vi "Teleop.vi"(10 "Match Info":T1={"Autonomous Elapsed Seconds"=0.0, "TeleOp Elapsed Seconds"=0.0, "Disabled Elapsed Seconds"=0.0, "Visited Autonomous"=FALSE, "Visited TeleOp"=FALSE, "Visited Disabled"=FALSE, "Autonomous Settings"={"Autonomous Style"=enum."Independent", "VI Refnum"=refnum}}, 11 "Call Context":T2) -> ()   [LabVIEW 2012]
doc: "This VI is called for each TeleOp packet received from the DS where the robot is not disabled. It is often used to read from the joysticks and update I/O or to update setpoints for timed control loops. It should complete and return within 20 milliseconds or it may miss DS packets."
uses:
  <vilib>/Rock Robotics/WPI/DriverStation/WPI_DriverStationDerivedRobotMode.ctl
  <vilib>/Rock Robotics/WPI/DriverStation/WPI_DriverStationMatch Info.ctl
  Robot Global Data.vi
  <vilib>/Rock Robotics/WPI/Joystick/WPI_JoystickGetSetRefNum.vi
  <vilib>/Rock Robotics/WPI/RobotDrive/WPI_RobotDriveGetSetRefNum.vi
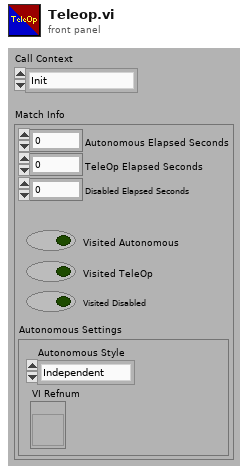
[diagram p1: front panel]
types:
  T1 = typedef "WPI_DriverStationMatch Info.ctl" = cluster{"Autonomous Elapsed Seconds":dbl, "TeleOp Elapsed Seconds":dbl, "Disabled Elapsed Seconds":dbl, "Visited Autonomous":bool, "Visited TeleOp":bool, "Visited Disabled":bool, "Autonomous Settings":cluster{"Autonomous Style":enum16{"Iterative", "Independent"}, "VI Refnum":refnum<vi>}}
  T2 = typedef "WPI_DriverStationDerivedRobotMode.ctl" = enum16{"Init", "Execute", "Stop"}
  T3 = typedef "WPI_DigitalInputDevRef.ctl" = cluster{"DevStatus":errorcluster, "DIO Channel":T4, "Digital Module":T5}
  T4 = typedef "FPGA_DIOChannel.ctl" = enum8{"DIO 1", "DIO 2", "DIO 3", "DIO 4", "DIO 5", "DIO 6", "DIO 7", "DIO 8", "DIO 9", "DIO 10", "DIO 11", "DIO 12", "DIO 13", "DIO 14", "Invalid"}
  T5 = typedef "FPGA_TypedefDigitalModule.ctl" = enum16{"Digital Module 1", "Digital Module 2"}
  T6 = cluster{"Prox1":bool, "Prox2":bool, "Prox3":bool, "Frisbee_Catch":bool, "Frisbee_Side_Check":bool, "Shooter_Ready":bool, "LeadScrewEnd":bool}
  T7 = typedef "WPI_JoystickDevRef.ctl" = cluster{"Device":T8}
  T8 = typedef "WPI_JoystickDeviceEnum.ctl" = enum16{"USB 1", "USB 2", "USB 3", "USB 4", "Kinect 1", "Kinect 2"}
  T9 = typedef "WPI_JoystickButtonState.ctl" = cluster{"Button 1":bool, "Button 2":bool, "Button 3":bool, "Button 4":bool, "Button 5":bool, "Button 6":bool, "Button 7":bool, "Button 8":bool, "Button 9":bool, "Button 10":bool, "Button 11":bool, "Button 12":bool}
  T10 = cluster{"axis 1 (x)":dbl, "axis 2 (y)":dbl, "axis 3 (throttle)":dbl, "axis 4":dbl, "axis 5":dbl, "axis 6":dbl}
  T11 = typedef "WPI_RobotDriveDevRef.ctl" = cluster{"DevStatus":errorcluster, "Motors[]":T12[], "Square Inputs":bool, "Max Output":dbl, "Isochronous":bool}
  T12 = typedef "WPI_MotorControlDeviceRef.ctl" = cluster{"DeviceStatus":errorcluster, "Type":enum16{"PWM", "CAN"}, "PWM":cluster{"Digital Module":T5, "PWM Channel":T13, "DeadBand":T14}, "CAN":cluster{"Device Number":u8, "Control Mode":T15, "Semaphore":T16, "Max Vout":dbl}, "Invert":bool, "TransformRef":T17, "InvTransformRef":T17}
  T13 = typedef "FPGA_DIOPWMChannel.ctl" = enum8{"PWM 1", "PWM 2", "PWM 3", "PWM 4", "PWM 5", "PWM 6", "PWM 7", "PWM 8", "PWM 9", "PWM 10", "Invalid"}
  T14 = typedef "WPI_PWMDeadband.ctl" = cluster{"Name":string, "maxPositivePwm":i32, "minPositivePwm":i32, "centerPwm":i32, "maxNegativePwm":i32, "minNegativePwm":i32, "angularRange":u16}
  T15 = typedef "WPI_CANJaguar_ControlMode.ctl" = enum8{"Percent VBus", "Current", "Speed", "Position", "Voltage"}
  T16 = typedef "Semaphore RefNum" = refnum<k1>
  T17 = typedef "WPI_PWMTransform_ConPane.ctl" = refnum<vi>
  T18 = cluster{"Shoot":bool, "Enable_Targeting":bool, "Shooter":dbl, "LeadScrew":dbl, "Feed":bool, "SuctionCup":bool, "SuctionRotate":bool, "SuctionExtend":bool, "Pickup":bool, "PizzaBottom":bool, "PizzaMid":bool, "Pizza_top":bool}
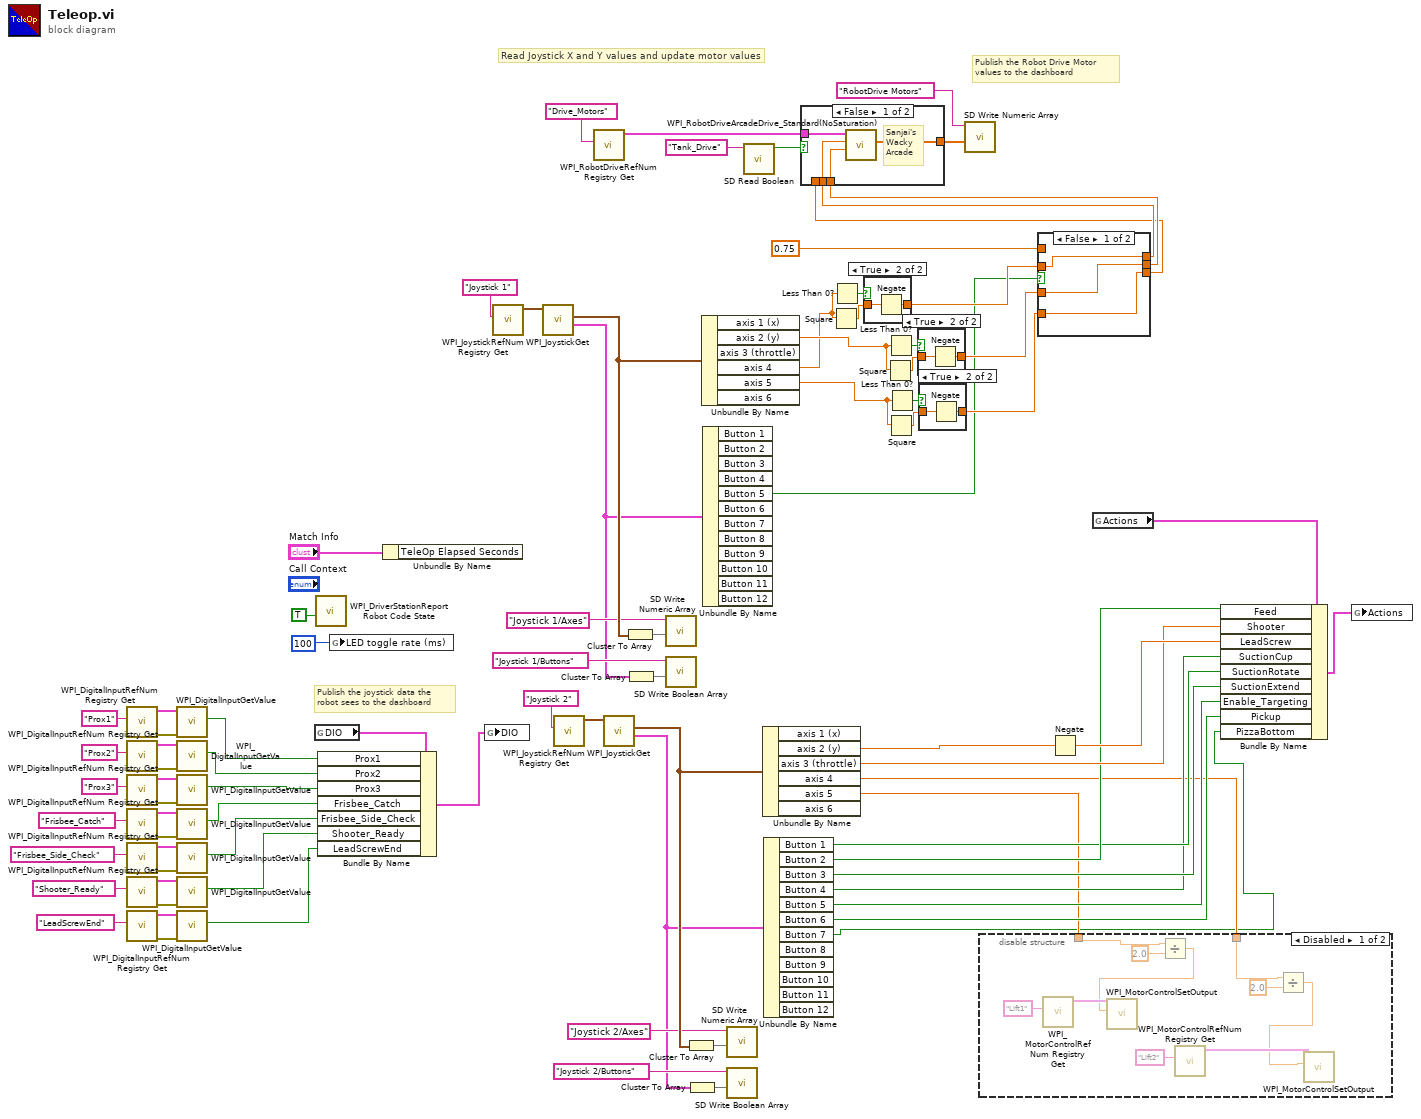
[diagram p0: block diagram]
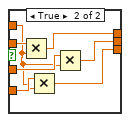
[diagram p3: hidden frame]
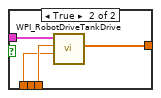
[diagram p7: hidden frame]
diagram:
  # "Publish the Robot Drive Motor\nvalues to the dashboard"
  # "Publish the joystick data the\nrobot sees to the dashboard"
  # "Read Joystick X and Y values and update motor values"
  n1 = call <vilib>:"WPI_DigitalInputRefNum Registry Get.vi"("refnum name"="Prox1") -> ("error out"=w61:errorcluster, "DigitalInputDevRef"=w60:T3)  [unwired: 9 in]
  n2 = call <vilib>:"WPI_DigitalInputRefNum Registry Get.vi"("refnum name"="Prox2") -> ("error out"=w52:errorcluster, "DigitalInputDevRef"=w53:T3)  [unwired: 9 in]
  n3 = call <vilib>:"WPI_DigitalInputRefNum Registry Get.vi"("refnum name"="Prox3") -> ("error out"=w51:errorcluster, "DigitalInputDevRef"=w54:T3)  [unwired: 9 in]
  n4 = call <vilib>:"WPI_DigitalInputRefNum Registry Get.vi"("refnum name"="Frisbee_Catch") -> ("error out"=w50:errorcluster, "DigitalInputDevRef"=w55:T3)  [unwired: 9 in]
  n5 = call <vilib>:"WPI_DigitalInputRefNum Registry Get.vi"("refnum name"="Frisbee_Side_Check") -> ("error out"=w57:errorcluster, "DigitalInputDevRef"=w56:T3)  [unwired: 9 in]
  n6 = call <vilib>:"WPI_DigitalInputRefNum Registry Get.vi"("refnum name"="Shooter_Ready") -> ("error out"=w59:errorcluster, "DigitalInputDevRef"=w58:T3)  [unwired: 9 in]
  n7 = call <vilib>:"WPI_DigitalInputRefNum Registry Get.vi"("refnum name"="LeadScrewEnd") -> ("error out"=w17:errorcluster, "DigitalInputDevRef"=w16:T3)  [unwired: 9 in]
  n8 = call <vilib>:"WPI_DigitalInputGetValue.vi"("error in (no error)"=w61, "DigitalInputDevRef"=w60) -> ("Value"=w44:bool)  [unwired: 7 in, 2 out]
  n9 = call <vilib>:"WPI_DigitalInputGetValue.vi"("error in (no error)"=w52, "DigitalInputDevRef"=w53) -> ("Value"=w49:bool)  [unwired: 7 in, 2 out]
  n10 = call <vilib>:"WPI_DigitalInputGetValue.vi"("error in (no error)"=w51, "DigitalInputDevRef"=w54) -> ("Value"=w48:bool)  [unwired: 7 in, 2 out]
  n11 = call <vilib>:"WPI_DigitalInputGetValue.vi"("error in (no error)"=w50, "DigitalInputDevRef"=w55) -> ("Value"=w47:bool)  [unwired: 7 in, 2 out]
  n12 = call <vilib>:"WPI_DigitalInputGetValue.vi"("error in (no error)"=w57, "DigitalInputDevRef"=w56) -> ("Value"=w46:bool)  [unwired: 7 in, 2 out]
  n13 = call <vilib>:"WPI_DigitalInputGetValue.vi"("error in (no error)"=w59, "DigitalInputDevRef"=w58) -> ("Value"=w45:bool)  [unwired: 7 in, 2 out]
  n14 = call <vilib>:"WPI_DigitalInputGetValue.vi"("error in (no error)"=w17, "DigitalInputDevRef"=w16) -> ("Value"=w14:bool)  [unwired: 7 in, 2 out]
  n15 = global read "Robot Global Data.vi" "DIO"() -> (w69:T6)
  n16 = call <vilib>:"WPI_DriverStationReport Robot Code State.vi"("TeleOp"=TRUE ("Autonomous")) -> ()  [unwired: 10 in, 1 out]
  n17 = Bundle By Name(cluster=w69, "Prox1"=w44, "Prox2"=w49, "Prox3"=w48, "Frisbee_Catch"=w47, "Frisbee_Side_Check"=w46, "Shooter_Ready"=w45, "LeadScrewEnd"=w14) -> (w68:T6)
  n18 = global write "Robot Global Data.vi" "LED toggle rate (ms)"(u32 100 ("LED ms toggle rate")) -> ()
  n19 = Unbundle By Name("Match Info") -> ()  [unwired: 1 out]
  n20 = global write "Robot Global Data.vi" "DIO"(w68) -> ()
  n21 = call <vilib>:"WPI_JoystickRefNum Registry Get.vi"("refnum name"="Joystick 1") -> ("JoystickDevRef"=w81:T7)  [unwired: 1 in, 9 out]
  n22 = call <vilib>:"WPI_JoystickGet.vi"("JoystickDevRef"=w81) -> ("Buttons"=w71:T9, "Axes"=w78:T10)  [unwired: 1 in, 4 out]
  n23 = call <vilib>:"WPI_JoystickRefNum Registry Get.vi"("refnum name"="Joystick 2") -> ("JoystickDevRef"=w34:T7)  [unwired: 1 in, 9 out]
  n24 = call <vilib>:"WPI_RobotDriveRefNum Registry Get.vi"("refnum name"="Drive_Motors") -> ("RobotDriveDevRef"=w83:T11)  [unwired: 1 in, 9 out]
  n25 = call <vilib>:"WPI_JoystickGet.vi"("JoystickDevRef"=w34) -> ("Buttons"=w28:T9, "Axes"=w31:T10)  [unwired: 1 in, 4 out]
  n26 = Cluster To Array(cluster=w78) -> (array=w77:dbl[])
  n27 = Cluster To Array(cluster=w71) -> (array=w80:bool[])
  n28 = call <vilib>:"SD Write Numeric Array.vi"("Numeric Array"=w77, "Name"="Joystick 1/Axes") -> ()  [unwired: 8 in, 2 out]
  n29 = call <vilib>:"SD Write Boolean Array.vi"("Boolean Array"=w80, "Name"="Joystick 1/Buttons") -> ()  [unwired: 8 in, 2 out]
  n30 = Cluster To Array(cluster=w31) -> (array=w30:dbl[])
  n31 = Cluster To Array(cluster=w28) -> (array=w33:bool[])
  n32 = Unbundle By Name(w78) -> ("axis 2 (y)"=w39:dbl, "axis 4"=w36:dbl, "axis 5"=w35:dbl)  [unwired: 3 out]
  n33 = Unbundle By Name(w71) -> ("Button 5"=w19:bool)  [unwired: 11 out]
  n34 = call <vilib>:"SD Write Numeric Array.vi"("Numeric Array"=w30, "Name"="Joystick 2/Axes") -> ()  [unwired: 8 in, 2 out]
  n35 = call <vilib>:"SD Write Boolean Array.vi"("Boolean Array"=w33, "Name"="Joystick 2/Buttons") -> ()  [unwired: 8 in, 2 out]
  n36 = call <vilib>:"SD Read Boolean.vi"("Name"="Tank_Drive") -> ("Boolean"=w73:bool)  [unwired: 8 in, 2 out]
  n37 = Unbundle By Name(w31) -> ("axis 2 (y)"=w15:dbl, "axis 3 (throttle)"=w10:dbl, "axis 4"=w3:dbl, "axis 5"=w2:dbl)  [unwired: 2 out]
  n38 = Unbundle By Name(w28) -> ("Button 1"=w7:bool, "Button 2"=w9:bool, "Button 3"=w8:bool, "Button 4"=w6:bool, "Button 5"=w5:bool, "Button 6"=w4:bool, "Button 7"=w1:bool)  [unwired: 5 out]
  n39 = Square(x=w36) -> (x^2=w43:dbl)
  n40 = Less Than 0?(x=w36) -> (x < 0?=w42:bool)
  n41 = case shown="True" w42 {
    tunnel: [w87 w88] -> w24
    tunnel: w43 -> [w87 w89]
    frame False {
    }
    frame True {
      n42 = Negate(x=w89) -> (-x=w88:dbl)
    }
  }
  n43 = Square(x=w39) -> (x^2=w41:dbl)
  n44 = Less Than 0?(x=w39) -> (x < 0?=w40:bool)
  n45 = Square(x=w35) -> (x^2=w38:dbl)
  n46 = Less Than 0?(x=w35) -> (x < 0?=w37:bool)
  n47 = case shown="True" w40 {
    tunnel: [w90 w91] -> w26
    tunnel: w41 -> [w90 w92]
    frame False {
    }
    frame True {
      n48 = Negate(x=w92) -> (-x=w91:dbl)
    }
  }
  n49 = case shown="True" w37 {
    tunnel: [w93 w94] -> w25
    tunnel: w38 -> [w93 w95]
    frame False {
    }
    frame True {
      n50 = Negate(x=w95) -> (-x=w94:dbl)
    }
  }
  n51 = disable-structure shown="Disabled" {
    disable-tunnel: w3 -> [w101 _]
    disable-tunnel: w2 -> [w97 _]
    frame Disabled {
      n52 = call <vilib>:"WPI_MotorControlRefNum Registry Get.vi"("refnum name"="Lift1") -> ("MotorControlDevRef"=w105:T12)  [unwired: 9 in, 1 out]
      n53 = Divide(x=w97, y=2.0) -> (x/y=w96:dbl)
      n54 = call <vilib>:"WPI_MotorControlSetOutput.vi"("Output"=w96, "MotorControlDevRef"=w105) -> ()  [unwired: 7 in, 3 out]
      n55 = call <vilib>:"WPI_MotorControlRefNum Registry Get.vi"("refnum name"="Lift2") -> ("MotorControlDevRef"=w103:T12)  [unwired: 9 in, 1 out]
      n56 = Divide(x=w101, y=2.0) -> (x/y=w99:dbl)
      n57 = call <vilib>:"WPI_MotorControlSetOutput.vi"("Output"=w99, "MotorControlDevRef"=w103) -> ()  [unwired: 7 in, 3 out]
    }
    frame Enabled {
    }
  }
  n58 = case shown="False" w19 {
    tunnel: w26 -> [w106 w115]
    tunnel: w25 -> [w107 w114]
    tunnel: w24 -> [w108 w113]
    tunnel: [w108 w110] -> w22
    tunnel: [w106 w112] -> w23
    tunnel: [w107 w111] -> w21
    tunnel: 0.75 -> [_ w109]
    frame False {
    }
    frame True {
      n59 = Multiply(x=w113, y=w109) -> (x*y=w110:dbl)
      n60 = Multiply(x=w114, y=w109) -> (x*y=w111:dbl)
      n61 = Multiply(x=w115, y=w109) -> (x*y=w112:dbl)
    }
  }
  n62 = case shown="False" w73 {
    tunnel: w83 -> [w119 w122]
    tunnel: [w118 w123] -> w74
    tunnel: w22 -> [w117 _]
    tunnel: w23 -> [w116 w121]
    tunnel: w21 -> [_ w120]
    frame False {
      # "Sanjai's\nWacky\nArcade"
      n63 = call <vilib>:"WPI_RobotDriveArcadeDrive_Standard(NoSaturation).vi"("Y axis value"=w116, "X axis value"=w117, "RobotDriveDevRef"=w119) -> ("Motor Values"=w118:dbl[])  [unwired: 1 in, 7 out]
    }
    frame True {
      n64 = call <vilib>:"WPI_RobotDriveTankDrive.vi"("Right axis value"=w120, "Left axis value"=w121, "RobotDriveDevRef"=w122) -> ("Motor Values"=w123:dbl[])  [unwired: 6 in, 2 out]
    }
  }
  n65 = call <vilib>:"SD Write Numeric Array.vi"("Numeric Array"=w74, "Name"="RobotDrive Motors") -> ()  [unwired: 8 in, 2 out]
  n66 = Negate(x=w15) -> (-x=w11:dbl)
  n67 = global read "Robot Global Data.vi" "Actions"() -> (w13:T18)
  n68 = Bundle By Name(cluster=w13, "Feed"=w9, "Shooter"=w10, "LeadScrew"=w11, "SuctionCup"=w6, "SuctionRotate"=w7, "SuctionExtend"=w8, "Enable_Targeting"=w5, "Pickup"=w4, "PizzaBottom"=w1) -> (w12:T18)
  n69 = global write "Robot Global Data.vi" "Actions"(w12) -> ()
